vi "Get Target Names.vi"(8 "error in (no error)":errorcluster, 11 "Project Sync Tools in":refnum<class "Project Sync Tools.lvclass">) -> (0 "error out":errorcluster, 2 "Targets names":string[](array[string]), 3 "Project Sync Tools out":refnum<class "Project Sync Tools.lvclass">)   [LabVIEW 2019, in "Project Sync Tools.lvclass"]
uses:
  Project Sync Tools.lvclass
  Project Sync Tools.lvclass/Project Sync Tools.ctl
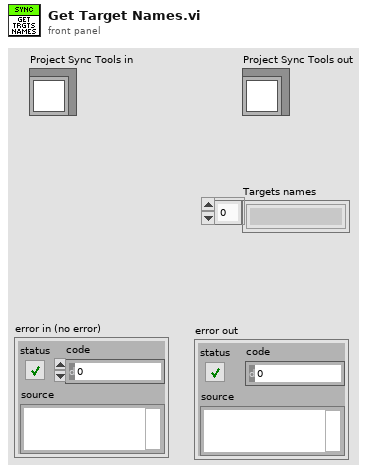
[diagram p1: front panel]
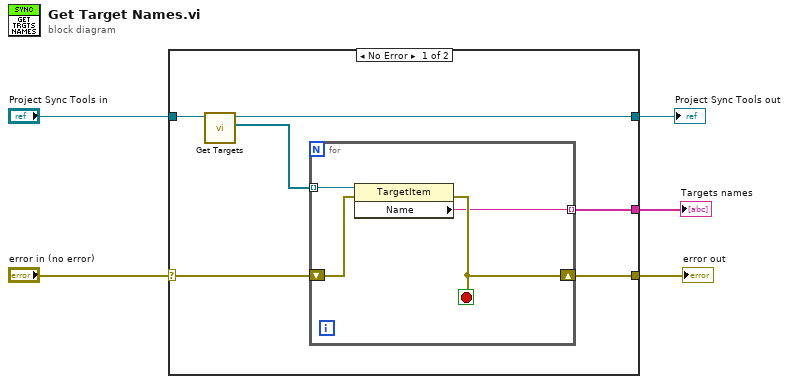
[diagram p0: block diagram]
diagram:
  n1 = case shown="No Error" "error in (no error)" {
    selector: "error in (no error)" -> [w7 w16]
    tunnel: [w11 w17] -> w5
    tunnel: "Project Sync Tools in" -> [w9 w17]
    tunnel: [w8 _] -> w3
    tunnel: [w6 w16] -> w1
    frame No Error {
      n2 = call "Get Targets.vi"("Project Sync Tools in"=w9) -> ("Targets"=w10:refnum<vi>[], "Project Sync Tools out"=w11:refnum<class "Project Sync Tools.lvclass">)  [unwired: 9 in]
      n3 = for {
        tunnel: w10 -> [w15] mode=indexing
        tunnel: [w12] -> w8 mode=indexing
        shift-right: [w13] -> w6
        shift-left: w7 -> [w14]
        stop <- w13 stop-if-true
        n4 = property class="TargetItem"(reference=w15, error in=w14) -> (error out=w13:errorcluster, "Name"=w12:string)  [unwired: 1 out]
      }
    }
    frame Error {
    }
  }
  "Project Sync Tools out" <- w5
  "Targets names" <- w3
  "error out" <- w1
